vi "begin stream read.vi"(5 "id":u32, 7 "event":refnum<user-event>, 8 "error in":errorcluster, 9 "max bytes":u32, 11 "socket":u64) -> (0 "error out":errorcluster)   [LabVIEW 2016, in "async tls.lvlib"]
uses:
  async tls.lvlib
  tls action complete user event.ctl
  lvasynctls.dll
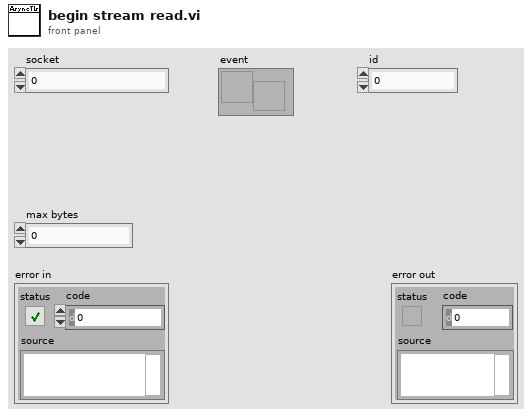
[diagram p1: front panel]
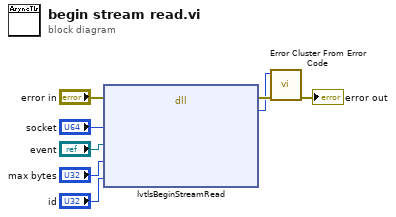
[diagram p0: block diagram]
diagram:
  n1 = dll-call lib="C:/Users/IEUser/Desktop/libasynclvtls/lvasynctls.dll" fn="lvtlsBeginStreamRead"(error in="error in", "socket"="socket", "event"="event", "bytes to read"="max bytes", "id"="id") -> (error out=w8:errorcluster, "err"=w7:i32)  [unwired: 6 in, 1 out]
  n2 = call <vilib>:"Error Cluster From Error Code.vi"("error in (no error)"=w8, "error code (0)"=w7) -> ("error out"=→"error out":errorcluster)  [unwired: 7 in]
